vi "SaveVariableToFile.vi"(11 "error in (no error)":errorcluster) -> (15 "error out":errorcluster)   [LabVIEW 2019, in "Stand.lvclass"]
uses:
  Stand.lvclass
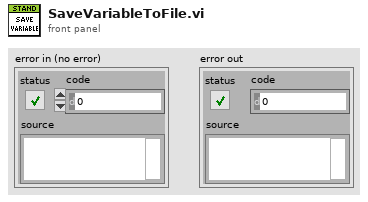
[diagram p1: front panel]
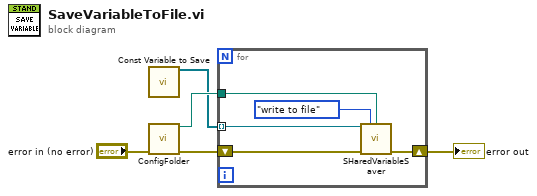
[diagram p0: block diagram]
diagram:
  n1 = call "Const Variable to Save.vi"() -> ("shared variable refnum out"=w1:refnum<k21>[])  [unwired: 15 in]
  n2 = call "ConfigFolder.vi"("error in (no error)"="error in (no error)") -> ("dup path"=w5:path, "error out"=w4:errorcluster)  [unwired: 13 in]
  n3 = for {
    shift-right: [w9] -> w2
    shift-left: w4 -> [w10]
    tunnel: w1 -> [w7] mode=indexing
    tunnel: w5 -> [w6]
    n4 = call "SHaredVariableSaver.vi"("shared variable refnum in"=w7, "cmd"=enum16{"read from file", "write to file"}."write to file", "dir"=w6, "error in (no error)"=w10) -> ("error out"=w9:errorcluster)  [unwired: 11 in]
  }
  "error out" <- w2
